vi "hwOperation_Verify License.vi"(0 "hwType":string, 3 "Error in":errorcluster) -> (10 "Error out":errorcluster)   [LabVIEW 2016]
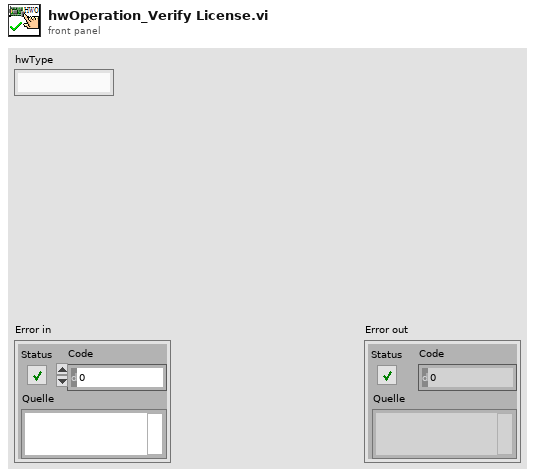
[diagram p1: front panel]
types:
  T1 = cluster{"TREE PNG":path, "User Guide":path, "DefaultSave":path, "BuildPath":path, "Image":path, "Modules":path, "Configuration":path, "License":path, "SplitFiles":path, "System.ini":path}
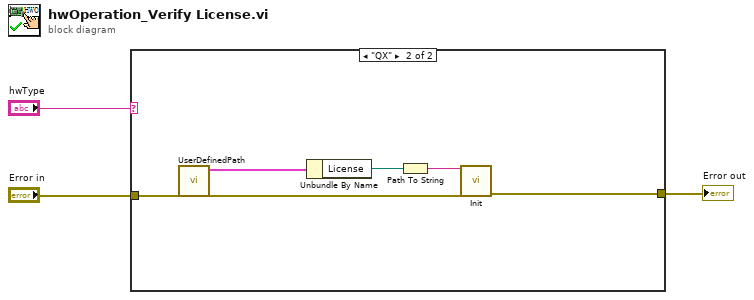
[diagram p0: block diagram]
diagram:
  n1 = case shown="\"QX\"" "hwType" {
    tunnel: "Error in" -> [w4 w6]
    tunnel: [w4 w5] -> w2
    frame "Simulation", Default {
    }
    frame "QX" {
      n2 = call "UserDefinedPath.vi"() -> ("UserDefinedPath"=w7:T1)  [unwired: 11 in]
      n3 = Unbundle By Name(w7) -> ("License"=w8:path)
      n4 = Path To String(path=w8) -> (string=w9:string)
      n5 = call "Init.vi"("LicenseFileName"=w9, "Error in"=w6) -> ("Error out"=w5:errorcluster)  [unwired: 6 in, 2 out]
    }
  }
  "Error out" <- w2
